vi "Edit.vi"(10 "TaskConfig":refnum<data-value>, 11 "TaskName":string) -> ()   [LabVIEW 2025, in "DAQ_Module.lvlib" / "DAQ_Module.lvclass"]
uses:
  DAQ_Module.lvclass
  DAQ_Task_Type.ctl
  DAQ_Linear_Task_Config.ctl
  DAQ_Angular_Task_Config.ctl
  DAQ_AI_Task_Config.ctl
  DAQ_HW_Type.ctl
  DAQ_SampleRateConfig.ctl
  DAQ_Config.ctl
  DAQ_Task_Config.ctl
  DAQ_Task_UIobject.ctl
  <vilib>/Utility/miscctls.llb/LVMapReplaceAction.ctl
  <vilib>/addons/_JKI Toolkits/State Machine/_JKI_lib_State_Machine.llb/Select State(s)_err__jki_lib_state_machine.vi
  DAQ_Module.lvclass/DAQ_Module.ctl
panel:
  in  "ShowPanel":bool
  in  "Enable":bool=TRUE
  in  "Cancel":bool
  in  "OK":bool
  in  "SampleRateConfiguration":T1={"SampleRate"=1000.0, "SamplesPerChannel"=1000, "SamplesPerRead"=200, "SampleMode"=10123, "Clock Source"="OnboardClock"} {"SampleMode" items=["Finite Samples"=10178, "Continuous Samples"=10123, "Hardware Timed Single Point"=12522]}
  in  "PhysicalChannels":string="/Dev1/ai0:3"
  in  "Drive":T2
  in  "TaskType":T3
  in  "Tab Control":enum32{"AI", "Linear", "Angular", "AO"}(tab)
  in  "AI_Config":T4={"MaxValue"=1.0, "MinValue"=0.0, "InputTerminalConfiguration"=-1} {"InputTerminalConfiguration" items=["default"=-1, "RSE"=10083, "NRSE"=10078, "Differential"=10106, "Pseudodifferential"=12529]}
  in  "LinearConfig":T5={"decoding type"=10092, "units"=10219, "distance per pulse"=0.001, "initial position"=0.0, "z index enable"=FALSE, "z index value"=0.0, "z index phase"=10040, "CI_Encoder_A_InputTerm"="", "CI_Encoder_B_InputTerm"="", "CI_Encoder_Z_InputTerm"=""} {"units" items=["Meters"=10219, "Inches"=10379, "Ticks"=10304, "From Custom Scale"=10065]; "decoding type" items=["X1"=10090, "X2"=10091, "X4"=10092, "Two Pulse Counting"=10313]; "z index phase" items=["A High B High"=10040, "A High B Low"=10041, "A Low B High"=10042, "A Low B Low"=10043]}
  in  "AngularConfig":T6={"decoding type"=10092, "units"=10146, "pulses per revolution"=24, "initial angle"=0.0, "z index enable"=FALSE, "z index value"=0.0, "z index phase"=10040, "CI_Encoder_A_InputTerm"="", "CI_Encoder_B_InputTerm"="", "CI_Encoder_Z_InputTerm"=""} {"units" items=["Degrees"=10146, "Radians"=10273, "Ticks"=10304, "From Custom Scale"=10065]; "decoding type" items=["X1"=10090, "X2"=10091, "X4"=10092, "Two Pulse Counting"=10313]; "z index phase" items=["A High B High"=10040, "A High B Low"=10041, "A Low B High"=10042, "A Low B Low"=10043]}
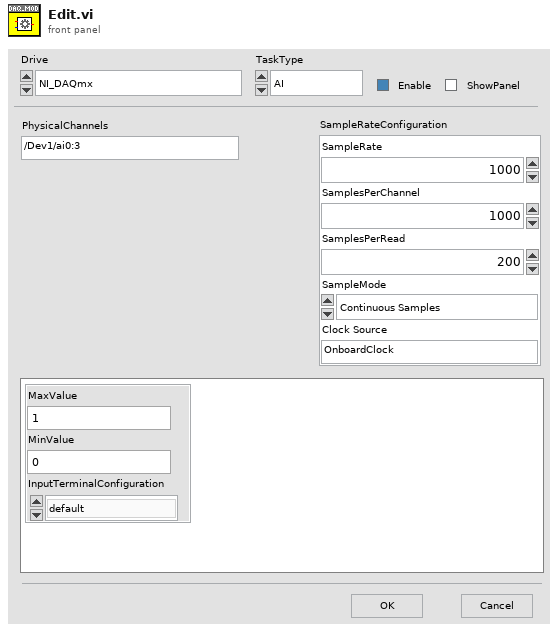
[diagram p1: front panel]
types:
  T1 = typedef "DAQ_Module.lvlib/DAQ_Module.lvclass/DAQ_SampleRateConfig.ctl" = cluster{"SampleRate":dbl, "SamplesPerChannel":u32, "SamplesPerRead":i32, "SampleMode":i32, "Clock Source":string}
  T2 = typedef "DAQ_Module.lvlib/DAQ_Module.lvclass/DAQ_HW_Type.ctl" = enum16{"NI_DAQmx", "Simulated_DAQ"}
  T3 = typedef "DAQ_Module.lvlib/DAQ_Module.lvclass/DAQ_Task_Type.ctl" = enum16{"AI", "Linear", "Angular", "AO"}
  T4 = typedef "DAQ_Module.lvlib/DAQ_Module.lvclass/DAQ_AI_Task_Config.ctl" = cluster{"MaxValue":dbl, "MinValue":dbl, "InputTerminalConfiguration":i32}
  T5 = typedef "DAQ_Module.lvlib/DAQ_Module.lvclass/DAQ_Linear_Task_Config.ctl" = cluster{"decoding type":i32, "units":i32, "distance per pulse":dbl, "initial position":dbl, "z index enable":bool, "z index value":dbl, "z index phase":i32, "CI_Encoder_A_InputTerm":string, "CI_Encoder_B_InputTerm":string, "CI_Encoder_Z_InputTerm":string}
  T6 = typedef "DAQ_Module.lvlib/DAQ_Module.lvclass/DAQ_Angular_Task_Config.ctl" = cluster{"decoding type":i32, "units":i32, "pulses per revolution":u32, "initial angle":dbl, "z index enable":bool, "z index value":dbl, "z index phase":i32, "CI_Encoder_A_InputTerm":string, "CI_Encoder_B_InputTerm":string, "CI_Encoder_Z_InputTerm":string}
  T7 = enum32{"Invalid", "Standard", "Closed", "Hidden", "Minimized", "Maximized"}
  T8 = enum32{"invalid app kind", "Development System", "Run Time System", "Student Edition", "Embedded LabVIEW", "Evaluation", "Custom"}
  T9 = typedef "LVMapReplaceAction.ctl" = enum32{"Modify Entry only if found", "Add or Modify Entry", "Delete Entry"}
  T10 = typedef "DAQ_Module.lvlib/DAQ_Module.lvclass/DAQ_Task_UIobject.ctl" = cluster{"Drive":refnum<vi>, "TaskType":refnum<vi>, "Enable":refnum<vi>, "PhysicalChannels":refnum<vi>, "SampleRateConfiguration":refnum<vi>, "AI_Config":refnum<vi>, "AngularConfig":refnum<vi>, "LinearConfig":refnum<vi>, "ShowPanel":refnum<vi>}
  T11 = cluster{"Core":cluster{"Current VI Reference":refnum<vi>, "Close Panel on Exit?":bool}, "Tab Control":refnum<vi>, "TaskConfig":refnum<data-value>, "TaskName":string, "Object":T10}
  T12 = cluster{"Current VI Reference":refnum<vi>, "Close Panel on Exit?":bool}
  T13 = typedef "DAQ_Module.lvlib/DAQ_Module.lvclass/DAQ_Config.ctl" = map{string, T14}
  T14 = typedef "DAQ_Module.lvlib/DAQ_Module.lvclass/DAQ_Task_Config.ctl" = cluster{"Drive":T2, "TaskType":T3, "PhysicalChannels":string, "SampleRateConfiguration":T1, "ChannelConfig":string, "Enable":bool, "ShowPanel":bool}
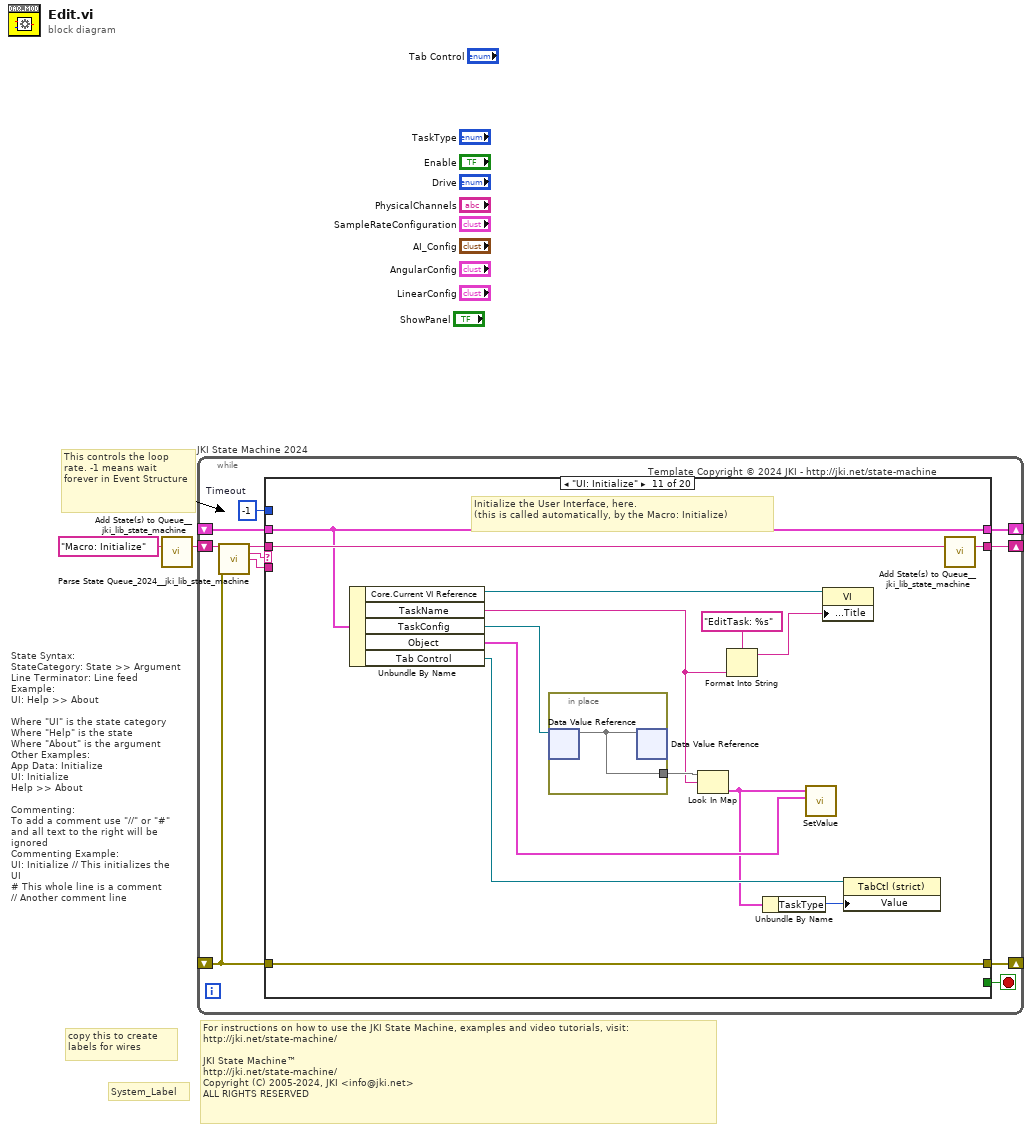
[diagram p0: block diagram]
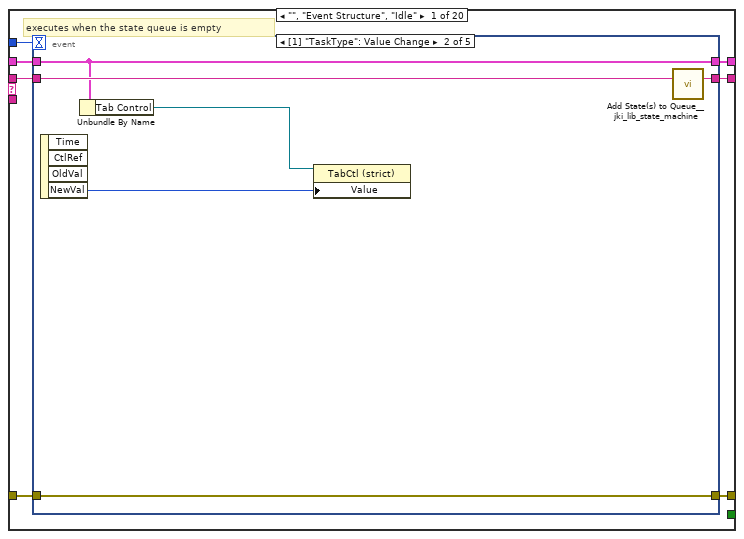
[diagram p2: hidden frame]
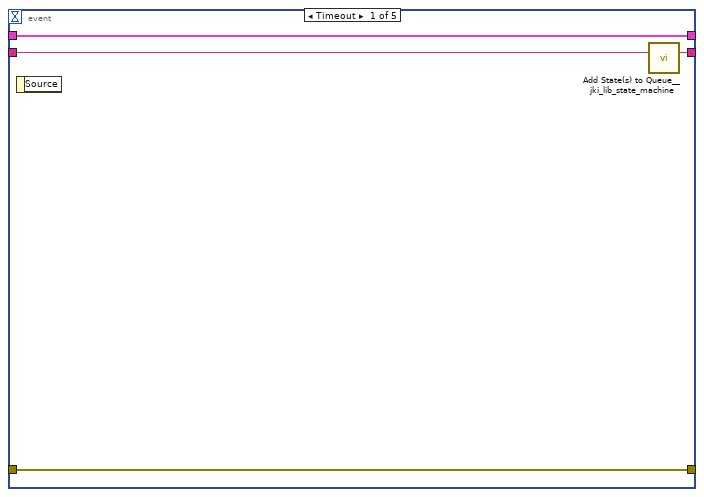
[diagram p3: hidden frame]
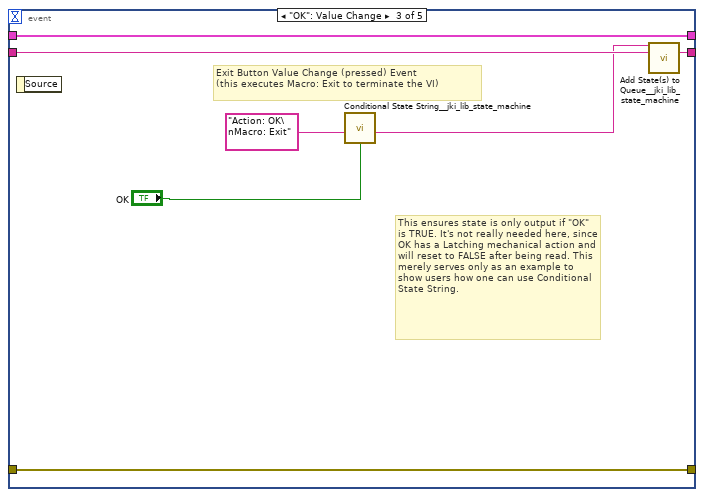
[diagram p4: hidden frame]
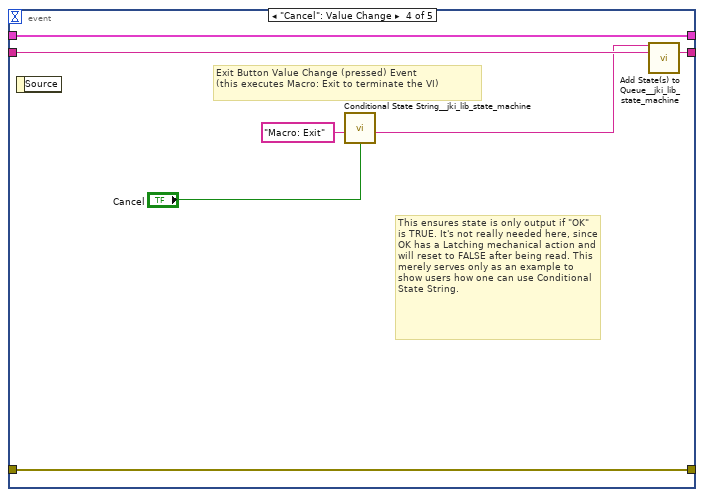
[diagram p5: hidden frame]
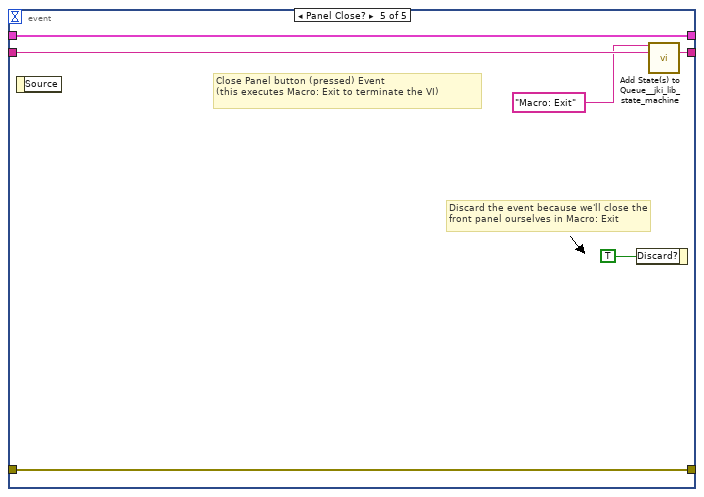
[diagram p6: hidden frame]
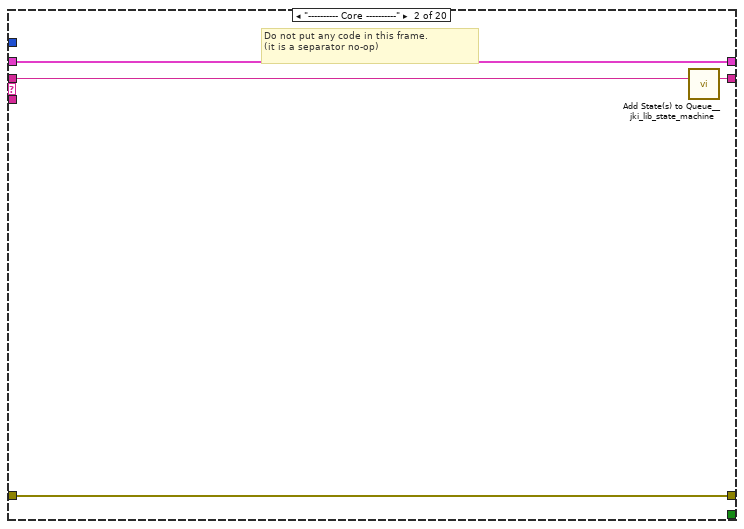
[diagram p7: hidden frame]
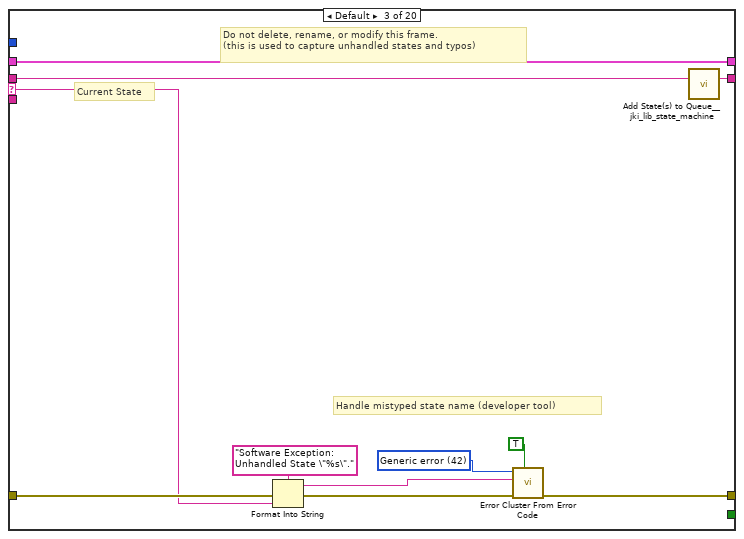
[diagram p8: hidden frame]
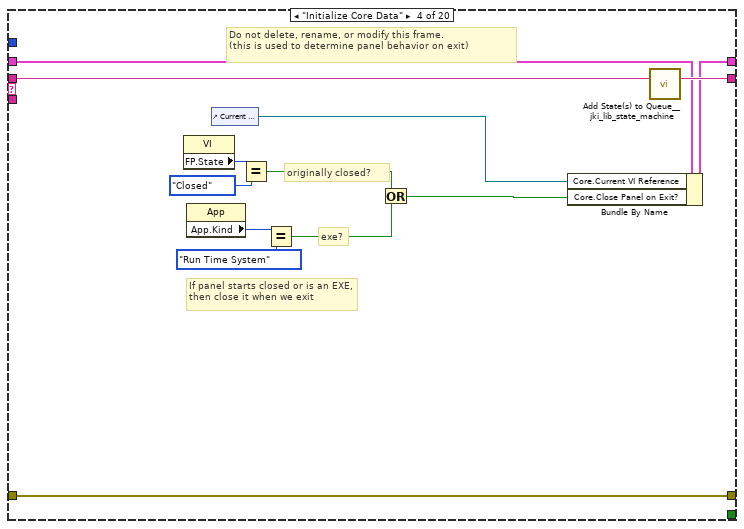
[diagram p9: hidden frame]
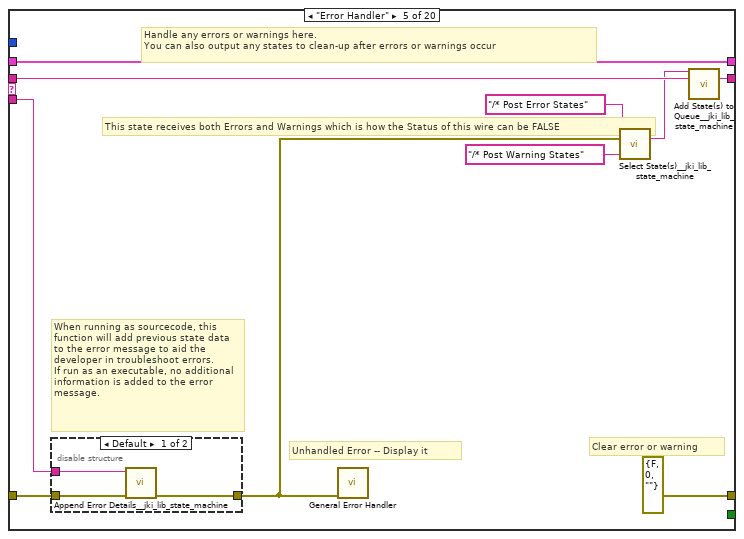
[diagram p10: hidden frame]
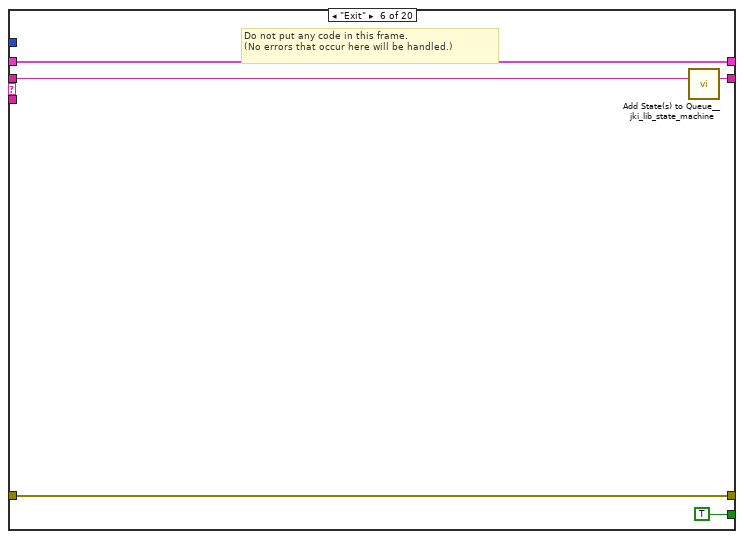
[diagram p12: hidden frame]
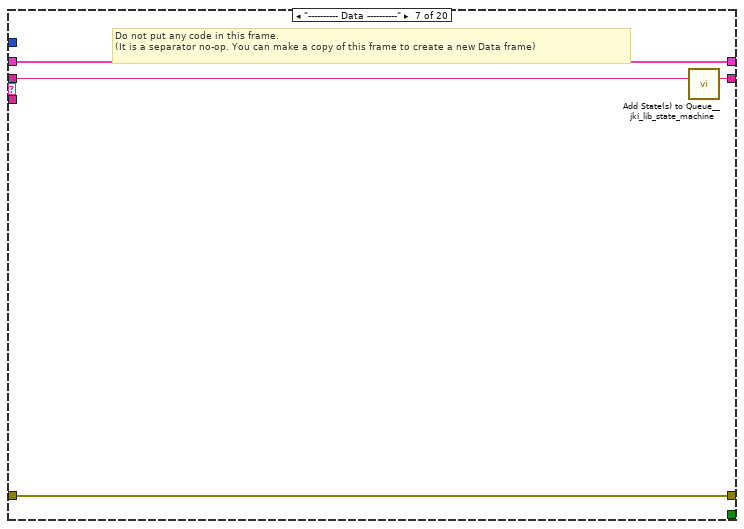
[diagram p13: hidden frame]
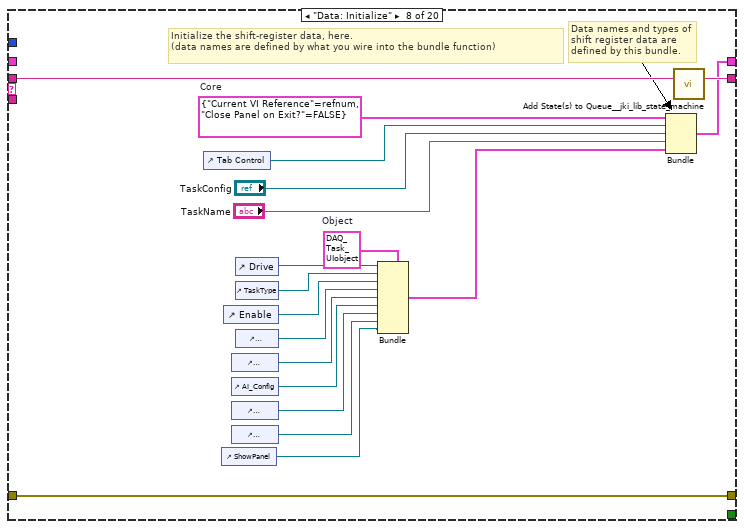
[diagram p14: hidden frame]
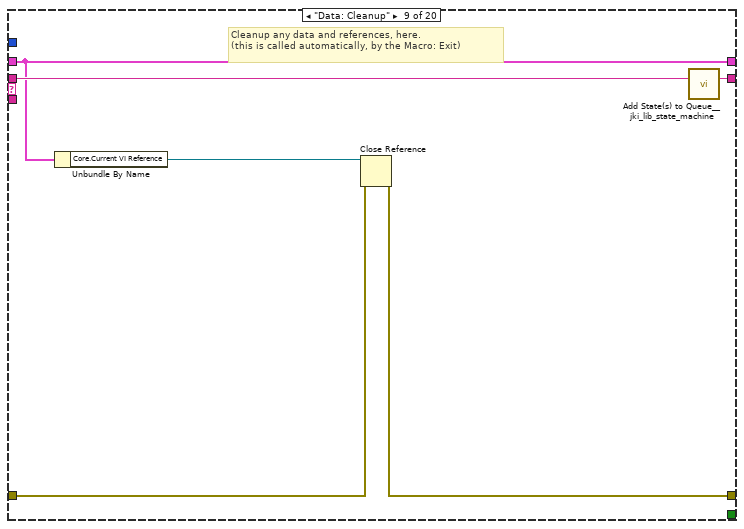
[diagram p15: hidden frame]
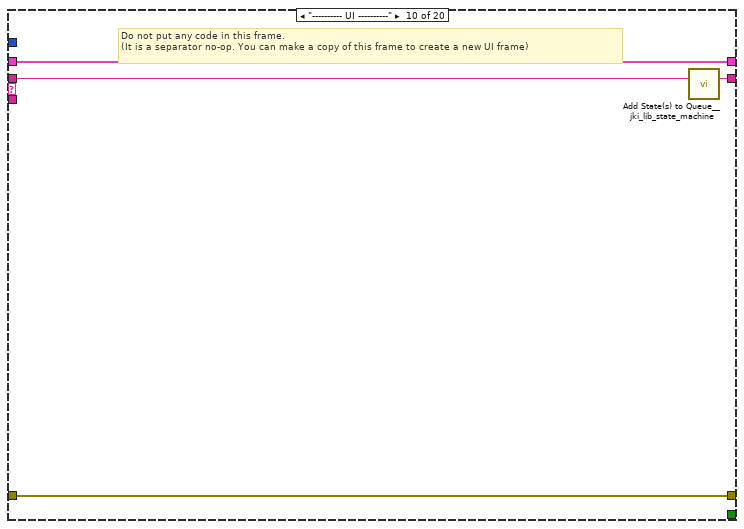
[diagram p16: hidden frame]
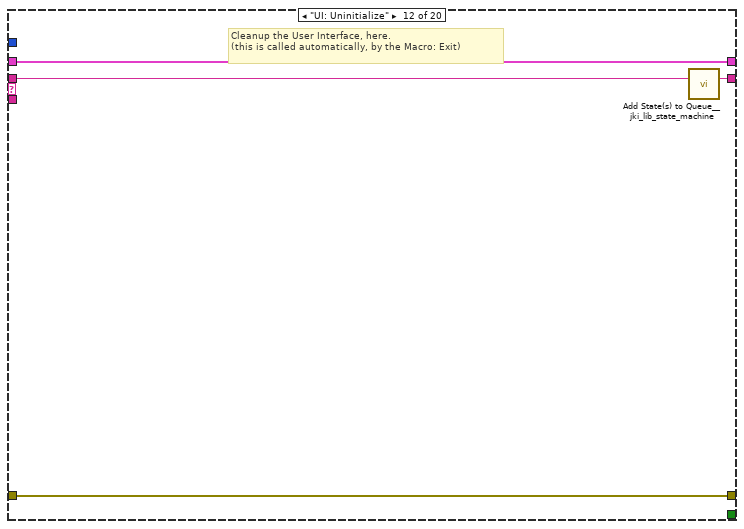
[diagram p17: hidden frame]
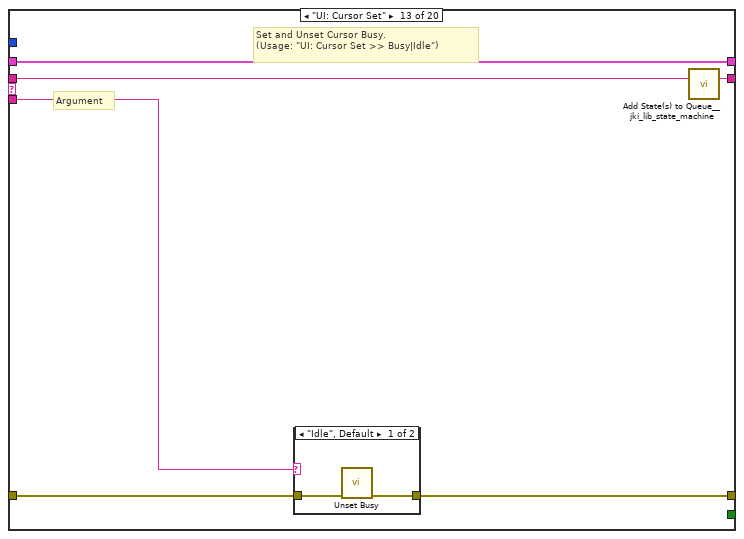
[diagram p18: hidden frame]
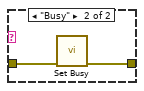
[diagram p19: hidden frame]
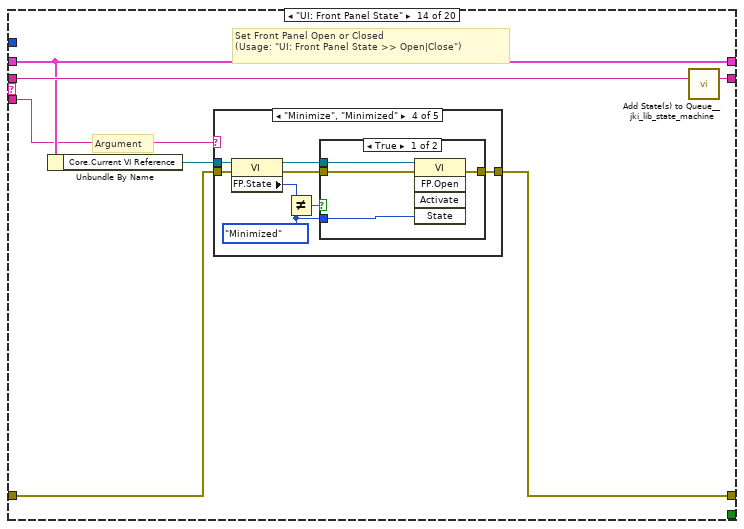
[diagram p20: hidden frame]
diagram:
  # "For instructions on how to use the JKI State Machine, examples and video tutorials, visit:\nhttp://jki.net/state-machine/\n\nJKI State Machine™\nhttp://jki.net/state-machine/\nCopyright (C) 2005-2024, JKI <info@jki.net>\nALL RIGHTS RESERVED"
  # "State Syntax:\nStateCategory: State >> Argument\nLine Terminator: Line feed\nExample:\nUI: Help >> About\n\nWhere \"UI\" is the state category\nWhere \"Help\" is the state\nWhere \"About\" is the argument\nOther Examples:\nApp Data: Initialize\nUI: Initialize\nHelp >> About\n\nCommenting:\nTo add a comment use \"//\" or \"#\" and all text to the right will be ignored\nCommenting Example:\nUI: Initialize // This initializes the UI\n# This whole line is a comment\n// Another comment line"
  # "copy this to create labels for wires"
  # "This controls the loop rate. -1 means wait forever in Event Structure"
  # "System_Label"
  n1 = call <vilib>:"Add State(s) to Queue__jki_lib_state_machine.vi"("State(s) in (\"\")"="Macro: Initialize") -> ("States Out"=w2:string)  [unwired: 14 in]
  n2 = while "JKI State Machine 2024" {
    shift-right: [w6] -> _
    shift-left: _ -> [w5]
    shift-right: [w9] -> _
    shift-left: _ -> [w3]
    shift-right: [w8] -> _
    shift-left: w2 -> [w10]
    stop <- w7 stop-if-true
    w4 = -1  # Timeout
    # "Template Copyright © 2024 JKI - http://jki.net/state-machine"
    n3 = call <vilib>:"Parse State Queue_2024__jki_lib_state_machine.vi"("State Queue"=w10, "Error In (no error)"=w3) -> ("Remaining States"=w12:string, "Current State"=w13:string, "Arguments"=w11:string)  [unwired: 11 in]
    n4 = case shown="\"UI: Initialize\"" w13 {
      selector: w13 -> [_ _ w55 _ _ _ _ _ _ _ _ _ _ _ _ _ _ _ _ _]
      tunnel: w12 -> [w20 w54 w59 w78 w88 w97 w101 w120 w126 w130 w144 w149 w155 w166 w235 w240 w249 w253 w261 w271]
      tunnel: w11 -> [_ _ _ _ w83 _ _ _ _ _ _ _ w150 w160 _ _ _ _ _ _]
      tunnel: w5 -> [w18 w51 w57 w71 w85 w95 w98 _ w121 w127 w141 w147 w153 w162 w232 w237 w247 w250 w258 w268]
      tunnel: [w17 w52 w61 w75 errorcluster {"status"=FALSE, "code"=0, "source"=""} ("error out") w94 w99 w117 w122 w128 w142 w146 w151 w163 w233 w238 w244 w251 w259 w269] -> w9
      tunnel: w3 -> [w14 w52 w60 w75 w84 w94 w99 w117 w123 w128 w142 w146 w152 w164 w233 w238 w244 w251 w259 w269]
      tunnel: [w19 w53 w58 w77 w87 w96 w100 w119 w125 w129 w143 w148 w154 w165 w234 w239 w248 w252 w260 w270] -> w8
      tunnel: [_ _ _ _ _ TRUE _ _ _ _ _ _ _ _ _ _ _ _ _ _] -> w7
      tunnel: [w16 w51 w57 w76 w85 w95 w98 w118 w121 w127 w141 w147 w153 w162 w232 w237 w247 w250 w258 w268] -> w6
      tunnel: w4 -> [w15 _ _ _ _ _ _ _ _ _ _ _ _ _ _ _ _ _ _ _]
      frame "", "Event Structure", "Idle" {
        # "executes when the state queue is empty"
        n5 = event shown="[1] \"TaskType\": Value Change" {
          selector: _ -> [_ _ _ _ _]
          dyn-events: _ -> [_ _ _ _ _]
          timeout: w15 -> [_ _ _ _ _]
          tunnel: w20 -> [w24 w30 w37 w44 w50]
          tunnel: [w23 w29 w36 w43 w49] -> w19
          tunnel: w18 -> [w21 w27 w34 w41 w47]
          tunnel: [w22 w28 w35 w42 w48] -> w17
          tunnel: w14 -> [w22 w28 w35 w42 w48]
          tunnel: [w21 w27 w34 w41 w47] -> w16
          event Timeout {
            n6 = event-data() -> ()  [unwired: 1 in, 1 out]
            n7 = call <vilib>:"Add State(s) to Queue__jki_lib_state_machine.vi"("State(s) in (\"\")"=w24) -> ("States Out"=w23:string)  [unwired: 14 in]
          }
          event Value Change {
            n8 = event-data() -> ("NewVal"=w25:T3)  [unwired: 1 in, 3 out]
            n9 = Unbundle By Name(w27) -> ("Tab Control"=w26:refnum<vi>)
            n10 = property class="TabCtl (strict)"(reference=w26, "Value"=w25) -> ()  [unwired: 1 in, 2 out]
            n11 = call <vilib>:"Add State(s) to Queue__jki_lib_state_machine.vi"("State(s) in (\"\")"=w30) -> ("States Out"=w29:string)  [unwired: 14 in]
          }
          event "OK": Value Change {
            # "This ensures state is only output if \"OK\" is TRUE. It's not really needed here, since OK has a Latching mechanical action and will reset to FALSE after being read. This merely serves only as an example to show users how one can use Conditional State String."
            # "Exit Button Value Change (pressed) Event\n(this executes Macro: Exit to terminate the VI)"
            n12 = event-data() -> ()  [unwired: 1 in, 1 out]
            n13 = call <vilib>:"Conditional State String__jki_lib_state_machine.vi"("Do State(s)?"="OK", "State"="Action: OK\nMacro: Exit") -> ("State Out"=w32:string)  [unwired: 7 in]
            n14 = call <vilib>:"Add State(s) to Queue__jki_lib_state_machine.vi"("State(s) in Front (\"\")"=w32, "State(s) in (\"\")"=w37) -> ("States Out"=w36:string)  [unwired: 13 in]
          }
          event "Cancel": Value Change {
            # "This ensures state is only output if \"OK\" is TRUE. It's not really needed here, since OK has a Latching mechanical action and will reset to FALSE after being read. This merely serves only as an example to show users how one can use Conditional State String."
            # "Exit Button Value Change (pressed) Event\n(this executes Macro: Exit to terminate the VI)"
            n15 = event-data() -> ()  [unwired: 1 in, 1 out]
            n16 = call <vilib>:"Conditional State String__jki_lib_state_machine.vi"("Do State(s)?"="Cancel", "State"="Macro: Exit") -> ("State Out"=w39:string)  [unwired: 7 in]
            n17 = call <vilib>:"Add State(s) to Queue__jki_lib_state_machine.vi"("State(s) in Front (\"\")"=w39, "State(s) in (\"\")"=w44) -> ("States Out"=w43:string)  [unwired: 13 in]
          }
          event Panel Close? {
            # "Discard the event because we'll close the front panel ourselves in Macro: Exit"
            # "Close Panel button (pressed) Event\n(this executes Macro: Exit to terminate the VI)"
            n18 = event-data() -> ()  [unwired: 1 in, 1 out]
            n19 = event-data("Discard?"=TRUE) -> ()  [unwired: 1 in, 1 out]
            n20 = call <vilib>:"Add State(s) to Queue__jki_lib_state_machine.vi"("State(s) in Front (\"\")"="Macro: Exit", "State(s) in (\"\")"=w50) -> ("States Out"=w49:string)  [unwired: 13 in]
          }
        }
      }
      frame "---------- Core ----------" {
        # "Do not put any code in this frame.\n(it is a separator no-op)"
        n21 = call <vilib>:"Add State(s) to Queue__jki_lib_state_machine.vi"("State(s) in (\"\")"=w54) -> ("States Out"=w53:string)  [unwired: 14 in]
      }
      frame Default {
        w64 = 42 items=["No error", "Argument error", "Memory is full", "Out of zone", "End of file", "File already open", "Generic file I/O error", "File not found", "File permission error", "Disk is full", "Duplicate path", "Too many files open", "System feature not enabled", "Resource file not found", "Cannot add resource", "Resource not found", "Image not found", "Image memory error", "Pen does not exist", "Config type invalid", "Config token not found", "Config parse error", "Config memory error", "Bad external code format", "Bad external code offset", "External code not present", "Null window", "Destroy window error", "Null menu", "Print aborted", "Bad print record", "Print driver error", "Windows error during printing", "Memory error during printing", "Print dialog error", "Generic print error", "Invalid device refnum", "Device not found", "Device parameter error", "Device unit error", "Cannot open device", "Device call aborted", "Generic error", "Cancelled by user", "Object ID too low", "Object ID too high", "Object not in heap", "Unknown heap", "Unknown object (invalid DefProc)", "Unknown object (DefProc not in table)", "Message out of range", "Invalid (null) method", "Unknown message", "Manager call not supported", "Bad address", "Network operation in progress", "Network operation timed out", "Connection is busy", "Network attribute not supported", "Network error", "Address in use", "System out of memory", "Connection aborted", "Connection refused", "Not connected", "Already connected", "Connection closed", "Initialization error (interapplication manager)", "Bad occurrence", "Wait on unbound occurrence handler", "Occurrence queue overflow", "Datalog type conflict", "Unused", "Unrecognized type (interapplication manager)", "Memory corrupt", "Failed to make temporary DLL", "Old CIN version", "Drag socket not found", "Failed to load drop-object", "Failed to register OLE object", "Failed to release OLE object", "Format specifier type mismatch", "Unknown format specifier", "Too few format specifiers", "Too many format specifiers", "Scan failed", "Newer CIN version", "Error converting to variant", "Runtime menu error", "Password tampered", "Variant attribute not found", "Incompatible variant data type", "Event data is not available", "Event Store is not present", "Occurrence is not found", "Event Queue is not created", "Event info is not available", "Refnum passed is NULL", "Error retrieving Class GUID", "Error retrieving CoClass GUID", "Error retrieving TypeLib GUID.", "Bad built application magic bytes.", "Specific driver is different from the specific driver associated with the Logical Name.", "There is no session opened to the class driver.", "Max Error", "MAX - Error with config objects", "MAX - Error loading configuration", "MAX - Group not supported"]
        # "Current State"
        # "Do not delete, rename, or modify this frame.\n(this is used to capture unhandled states and typos)"
        # "Handle mistyped state name (developer tool)"
        n22 = Format Into String(format string="Software Exception: Unhandled State \"%s\"." ("message"), error in=w60, w55) -> (resulting string=w63:string, error out=w62:errorcluster)  [unwired: 1 in]
        n23 = call <vilib>:"Error Cluster From Error Code.vi"("show call chain? (False)"=TRUE, "error in (no error)"=w62, "error message (\"\")"=w63, "error code (0)"=w64) -> ("error out"=w61:errorcluster)  [unwired: 5 in]
        n24 = call <vilib>:"Add State(s) to Queue__jki_lib_state_machine.vi"("State(s) in (\"\")"=w59) -> ("States Out"=w58:string)  [unwired: 14 in]
      }
      frame "Initialize Core Data" {
        # "Do not delete, rename, or modify this frame.\n(this is used to determine panel behavior on exit)"
        # "originally closed?"
        # "exe?"
        # "If panel starts closed or is an EXE, then close it when we exit"
        n25 = property class="VI"() -> ("FP.State"=w68:T7)  [unwired: 2 in, 2 out]
        n26 = property class="App"() -> ("App.Kind"=w74:T8)  [unwired: 2 in, 2 out]
        n27 = control-ref of="Current VI Reference"() -> (w69:refnum<vi>)
        n28 = Equal?(x=w68, y=T7."Closed" ("Front Panel Window:State")) -> (x = y?=w66:bool)
        n29 = Equal?(x=w74, y=T8."Run Time System" ("Application:Kind")) -> (x = y?=w72:bool)
        n30 = Or(x=w66, y=w72) -> (x .or. y?=w70:bool)
        n31 = Bundle By Name(cluster=w71, "Core.Current VI Reference"=w69, "Core.Close Panel on Exit?"=w70) -> (w76:T11)
        n32 = call <vilib>:"Add State(s) to Queue__jki_lib_state_machine.vi"("State(s) in (\"\")"=w78) -> ("States Out"=w77:string)  [unwired: 14 in]
      }
      frame "Error Handler" {
        # "When running as sourcecode, this function will add previous state data to the error message to aid the developer in troubleshoot errors.\nIf run as an executable, no additional information is added to the error message."
        # "This state receives both Errors and Warnings which is how the Status of this wire can be FALSE"
        # "Unhandled Error -- Display it"
        # "Handle any errors or warnings here.\nYou can also output any states to clean-up after errors or warnings occur"
        # "Clear error or warning"
        n33 = disable-structure shown="Default" {
          disable-tunnel: w84 -> [w91 w92]
          disable-tunnel: w83 -> [w90 _]
          disable-tunnel: [w89 w92] -> w82
          frame condition #0 (active) {
            n34 = call <vilib>:"Append Error Details__jki_lib_state_machine.vi"("error in (no error)"=w91, "Previous State and Argument(s)"=w90) -> ("error out"=w89:errorcluster)  [unwired: 9 in]
          }
          frame condition #1 {
          }
        }
        n35 = call <vilib>:"General Error Handler.vi"("error in (no error)"=w82) -> ()  [unwired: 10 in, 5 out]
        n36 = call-poly <vilib>:"Select State(s)__jki_lib_state_machine.vi"("State(s) if True (\"\")"="/* Post Error States", "Select"=w82, "State(s) if False (\"\")"="/* Post Warning States") -> ("States Out"=w80:string)  [unwired: 12 in]
        n37 = call <vilib>:"Add State(s) to Queue__jki_lib_state_machine.vi"("State(s) in Front (\"\")"=w80, "State(s) in (\"\")"=w88) -> ("States Out"=w87:string)  [unwired: 13 in]
      }
      frame "Exit" {
        # "Do not put any code in this frame.\n(No errors that occur here will be handled.)"
        n38 = call <vilib>:"Add State(s) to Queue__jki_lib_state_machine.vi"("State(s) in (\"\")"=w97) -> ("States Out"=w96:string)  [unwired: 14 in]
      }
      frame "---------- Data ----------" {
        # "Do not put any code in this frame.\n(It is a separator no-op. You can make a copy of this frame to create a new Data frame)"
        n39 = call <vilib>:"Add State(s) to Queue__jki_lib_state_machine.vi"("State(s) in (\"\")"=w101) -> ("States Out"=w100:string)  [unwired: 14 in]
      }
      frame "Data: Initialize" {
        w103 = T10 {"Drive"=refnum, "TaskType"=refnum, "Enable"=refnum, "PhysicalChannels"=refnum, "SampleRateConfiguration"=refnum, "AI_Config"=refnum, "AngularConfig"=refnum, "LinearConfig"=refnum, "ShowPanel"=refnum}  # Object
        w116 = T12 {"Current VI Reference"=refnum, "Close Panel on Exit?"=FALSE}  # Core
        # "Data names and types of shift register data are defined by this bundle."
        # "Initialize the shift-register data, here.\n(data names are defined by what you wire into the bundle function)"
        n40 = control-ref of="Tab Control"() -> (w115:refnum<vi>)
        n41 = control-ref of="ShowPanel"() -> (w102:refnum<vi>)
        n42 = control-ref of="Enable"() -> (w110:refnum<vi>)
        n43 = control-ref of="SampleRateConfiguration"() -> (w108:refnum<vi>)
        n44 = control-ref of="AI_Config"() -> (w107:refnum<vi>)
        n45 = control-ref of="AngularConfig"() -> (w106:refnum<vi>)
        n46 = control-ref of="LinearConfig"() -> (w105:refnum<vi>)
        n47 = control-ref of="Drive"() -> (w112:refnum<vi>)
        n48 = control-ref of="TaskType"() -> (w111:refnum<vi>)
        n49 = control-ref of="PhysicalChannels"() -> (w109:refnum<vi>)
        n50 = Bundle(cluster=w103, "Drive"=w112, "TaskType"=w111, "Enable"=w110, "PhysicalChannels"=w109, "SampleRateConfiguration"=w108, "AI_Config"=w107, "AngularConfig"=w106, "LinearConfig"=w105, "ShowPanel"=w102) -> (w104:T10)
        n51 = Bundle("Core"=w116, "Tab Control"=w115, "TaskConfig"="TaskConfig", "TaskName"="TaskName", "Object"=w104) -> (w118:T11)  [unwired: 1 in]
        n52 = call <vilib>:"Add State(s) to Queue__jki_lib_state_machine.vi"("State(s) in (\"\")"=w120) -> ("States Out"=w119:string)  [unwired: 14 in]
      }
      frame "Data: Cleanup" {
        # "Cleanup any data and references, here.\n(this is called automatically, by the Macro: Exit)"
        n53 = Unbundle By Name(w121) -> ("Core.Current VI Reference"=w124:refnum<vi>)
        n54 = Close Reference(reference=w124, error in (no error)=w123) -> (error out=w122:errorcluster)
        n55 = call <vilib>:"Add State(s) to Queue__jki_lib_state_machine.vi"("State(s) in (\"\")"=w126) -> ("States Out"=w125:string)  [unwired: 14 in]
      }
      frame "---------- UI ----------" {
        # "Do not put any code in this frame.\n(It is a separator no-op. You can make a copy of this frame to create a new UI frame)"
        n56 = call <vilib>:"Add State(s) to Queue__jki_lib_state_machine.vi"("State(s) in (\"\")"=w130) -> ("States Out"=w129:string)  [unwired: 14 in]
      }
      frame "UI: Initialize" {
        # "Initialize the User Interface, here.\n(this is called automatically, by the Macro: Initialize)"
        n57 = Unbundle By Name(w141) -> ("Core.Current VI Reference"=w140:refnum<vi>, "TaskName"=w135:string, "TaskConfig"=w137:refnum<data-value>, "Object"=w134:T10, "Tab Control"=w133:refnum<vi>)
        n58 = in-place {
          in-place-border: [w145] -> w136
          n59 = in-place-dvr #1(w137) -> (w145:T13)  [unwired: 1 out]
          n60 = in-place-dvr #1(w145) -> ()  [unwired: 2 out]
        }
        n61 = Look In Map(map=w136, key=w135) -> (value=w132:T14)  [unwired: 1 in, 1 out]
        n62 = Format Into String(format string="EditTask: %s", w135) -> (resulting string=w138:string)  [unwired: 2 in, 1 out]
        n63 = Unbundle By Name(w132) -> ("TaskType"=w131:T3)
        n64 = call "SetValue.vi"("cluster"=w134, "TaskConfig"=w132) -> ()  [unwired: 10 in]
        n65 = property class="VI"(reference=w140, "Front Panel.Title"=w138) -> ()  [unwired: 1 in, 2 out]
        n66 = property class="TabCtl (strict)"(reference=w133, "Value"=w131) -> ()  [unwired: 1 in, 2 out]
        n67 = call <vilib>:"Add State(s) to Queue__jki_lib_state_machine.vi"("State(s) in (\"\")"=w144) -> ("States Out"=w143:string)  [unwired: 14 in]
      }
      frame "UI: Uninitialize" {
        # "Cleanup the User Interface, here.\n(this is called automatically, by the Macro: Exit)"
        n68 = call <vilib>:"Add State(s) to Queue__jki_lib_state_machine.vi"("State(s) in (\"\")"=w149) -> ("States Out"=w148:string)  [unwired: 14 in]
      }
      frame "UI: Cursor Set" {
        # "Argument"
        # "Set and Unset Cursor Busy.\n(Usage: \"UI: Cursor Set >> Busy|Idle\")"
        n69 = case shown="\"Idle\", Default" w150 {
          tunnel: w152 -> [w157 w159]
          tunnel: [w156 w158] -> w151
          frame "Idle", Default {
            n70 = call <vilib>:"Unset Busy.vi"("error in (no error)"=w157) -> ("error out"=w156:errorcluster)  [unwired: 10 in]
          }
          frame "Busy" {
            n71 = call <vilib>:"Set Busy.vi"("error in (no error)"=w159) -> ("error out"=w158:errorcluster)  [unwired: 9 in, 1 out]
          }
        }
        n72 = call <vilib>:"Add State(s) to Queue__jki_lib_state_machine.vi"("State(s) in (\"\")"=w155) -> ("States Out"=w154:string)  [unwired: 14 in]
      }
      frame "UI: Front Panel State" {
        # "Argument"
        # "Set Front Panel Open or Closed\n(Usage: \"UI: Front Panel State >> Open|Close\")"
        n73 = Unbundle By Name(w162) -> ("Core.Current VI Reference"=w161:refnum<vi>)
        n74 = case shown="\"Minimize\", \"Minimized\"" w160 {
          tunnel: w164 -> [w172 w187 w198 w211 w224]
          tunnel: [w174 w188 w200 w213 w226] -> w163
          tunnel: w161 -> [w173 w185 w199 w212 w225]
          frame "Open", "Standard", Default {
            w167 = T7."Standard" ("State")
            n75 = property class="VI"(reference=w173, error in=w172) -> (reference out=w170:refnum<vi>, error out=w171:errorcluster, "FP.State"=w169:T7)
            n76 = Not Equal?(x=w169, y=w167) -> (x != y?=w168:bool)
            n77 = case shown="True" w168 {
              tunnel: [w178 w180] -> w174
              tunnel: w171 -> [w177 w180]
              tunnel: w170 -> [w176 _]
              tunnel: w167 -> [w175 _]
              frame True {
                n78 = invoke class="VI" method="FP.Open"(reference=w176, error in=w177, "Activate"=TRUE, "State"=w175) -> (error out=w178:errorcluster)  [unwired: 1 in, 4 out]
              }
              frame False {
              }
            }
          }
          frame "Close", "Closed" {
            n79 = property class="VI"(reference=w185, error in=w187) -> (reference out=w184:refnum<vi>, error out=w186:errorcluster, "FP.State"=w182:T7)
            n80 = Not Equal?(x=w182, y=T7."Closed" ("Front Panel Window:State")) -> (x != y?=w181:bool)
            n81 = case shown="True" w181 {
              tunnel: [w189 w192] -> w188
              tunnel: w186 -> [w189 w191]
              tunnel: w184 -> [_ w190]
              frame False {
              }
              frame True {
                n82 = invoke class="VI" method="FP.Close"(reference=w190, error in=w191) -> (error out=w192:errorcluster)  [unwired: 1 in, 2 out]
              }
            }
          }
          frame "Hidden", "Hide" {
            w193 = T7."Hidden" ("State")
            n83 = property class="VI"(reference=w199, error in=w198) -> (reference out=w196:refnum<vi>, error out=w197:errorcluster, "FP.State"=w195:T7)
            n84 = Not Equal?(x=w195, y=w193) -> (x != y?=w194:bool)
            n85 = case shown="True" w194 {
              tunnel: [w204 w205] -> w200
              tunnel: w197 -> [w203 w205]
              tunnel: w196 -> [w202 _]
              tunnel: w193 -> [w201 _]
              frame True {
                n86 = invoke class="VI" method="FP.Open"(reference=w202, error in=w203, "State"=w201) -> (error out=w204:errorcluster)  [unwired: 2 in, 4 out]
              }
              frame False {
              }
            }
          }
          frame "Minimize", "Minimized" {
            w206 = T7."Minimized" ("State")
            n87 = property class="VI"(reference=w212, error in=w211) -> (reference out=w209:refnum<vi>, error out=w210:errorcluster, "FP.State"=w208:T7)
            n88 = Not Equal?(x=w208, y=w206) -> (x != y?=w207:bool)
            n89 = case shown="True" w207 {
              tunnel: [w217 w218] -> w213
              tunnel: w210 -> [w216 w218]
              tunnel: w209 -> [w215 _]
              tunnel: w206 -> [w214 _]
              frame True {
                n90 = invoke class="VI" method="FP.Open"(reference=w215, error in=w216, "State"=w214) -> (error out=w217:errorcluster)  [unwired: 2 in, 4 out]
              }
              frame False {
              }
            }
          }
          frame "Maximize", "Maximized" {
            w219 = T7."Maximized" ("State")
            n91 = property class="VI"(reference=w225, error in=w224) -> (reference out=w222:refnum<vi>, error out=w223:errorcluster, "FP.State"=w221:T7)
            n92 = Not Equal?(x=w221, y=w219) -> (x != y?=w220:bool)
            n93 = case shown="True" w220 {
              tunnel: [w230 w231] -> w226
              tunnel: w223 -> [w229 w231]
              tunnel: w222 -> [w228 _]
              tunnel: w219 -> [w227 _]
              frame True {
                n94 = invoke class="VI" method="FP.Open"(reference=w228, error in=w229, "State"=w227) -> (error out=w230:errorcluster)  [unwired: 2 in, 4 out]
              }
              frame False {
              }
            }
          }
        }
        n95 = call <vilib>:"Add State(s) to Queue__jki_lib_state_machine.vi"("State(s) in (\"\")"=w166) -> ("States Out"=w165:string)  [unwired: 14 in]
      }
      frame "---------- Macro ----------" {
        # "Do not put any code in this frame.\n(It is a separator no-op. You can make a copy of this frame to create a new Macro frame)"
        n96 = call <vilib>:"Add State(s) to Queue__jki_lib_state_machine.vi"("State(s) in (\"\")"=w235) -> ("States Out"=w234:string)  [unwired: 14 in]
      }
      frame "Macro: Initialize" {
        w236 = "Data: Initialize\nInitialize Core Data\nUI: Initialize\nUI: Front Panel State >> Open"  # Data: Initialize Initialize Core Data UI: Initialize UI: Front Panel State >> Open
        # "Initialization Macro\n(This is called once, when the VI starts)"
        n97 = call <vilib>:"Add State(s) to Queue__jki_lib_state_machine.vi"("State(s) in Front (\"\")"=w236, "State(s) in (\"\")"=w240) -> ("States Out"=w239:string)  [unwired: 13 in]
      }
      frame "Macro: Exit" {
        # "Exit Macro\n(This is called once, when the VI exits)"
        n98 = Unbundle By Name(w247) -> ("Core.Close Panel on Exit?"=w242:bool)
        n99 = call <vilib>:"Conditional State String__jki_lib_state_machine.vi"("Do State(s)?"=w242, "State"="UI: Front Panel State >> Close") -> ("State Out"=w241:string)  [unwired: 7 in]
        n100 = call <vilib>:"Add State(s) to Queue__jki_lib_state_machine.vi"("State(s) in (\"\")"=w241, "State(s) at Back (\"\")"="UI: Uninitialize\nData: Cleanup\nExit") -> ("States Out"=w245:string)  [unwired: 13 in]
        n101 = call <vilib>:"Add State(s) to Queue__jki_lib_state_machine.vi"("State(s) in Front (\"\")"=w245, "State(s) in (\"\")"=w249) -> ("States Out"=w248:string)  [unwired: 13 in]
      }
      frame "---------- Action ----------" {
        # "Template Separator\n(You can make a copy of, or modify, this frame)"
        n102 = call <vilib>:"Add State(s) to Queue__jki_lib_state_machine.vi"("State(s) in (\"\")"=w253) -> ("States Out"=w252:string)  [unwired: 14 in]
      }
      frame "Action: OK" {
        # "Your code here.\n(You can make a copy of, or modify, this frame)"
        n103 = Unbundle By Name(w258) -> ("TaskConfig"=w257:refnum<data-value>, "TaskName"=w256:string, "Object"=w255:T10)
        n104 = call "GetValue.vi"("cluster"=w255) -> ("output cluster"=w254:T14)  [unwired: 10 in]
        n105 = in-place {
          in-place-border: w256 -> [w264]
          in-place-border: w254 -> [w262]
          n106 = in-place-dvr #2(w257) -> (w265:T13)  [unwired: 1 out]
          n107 = in-place {
            in-place-border: w262 -> [w266]
            n108 = in-place-map #3(w265, w264) -> ()  [unwired: 1 in, 2 out]
            n109 = in-place-map #3(w266, LVMapReplaceAction."Modify Entry only if found" ("action")) -> (w263:T13)  [unwired: 2 out]
          }
          n110 = in-place-dvr #2(w263) -> ()  [unwired: 2 out]
        }
        n111 = call <vilib>:"Add State(s) to Queue__jki_lib_state_machine.vi"("State(s) in (\"\")"=w261) -> ("States Out"=w260:string)  [unwired: 14 in]
      }
      frame "Action: Cancel" {
        # "Your code here.\n(You can make a copy of, or modify, this frame)"
        n112 = call <vilib>:"Add State(s) to Queue__jki_lib_state_machine.vi"("State(s) in (\"\")"=w271) -> ("States Out"=w270:string)  [unwired: 14 in]
      }
    }
  }
